vi "rainbow palette array.vi"() -> (0 "rainbow array":u32[](array[numeric]))   [LabVIEW 2009]
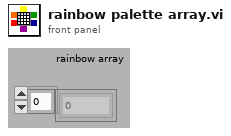
[diagram p1: front panel]
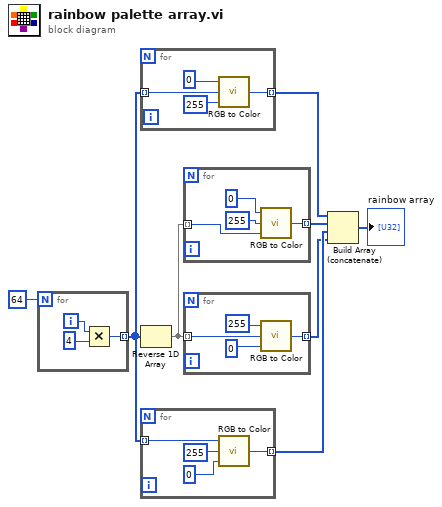
[diagram p0: block diagram]
diagram:
  n1 = for {
    N: 64 -> [_]
    tunnel: [w9] -> w7 mode=indexing
    i -> [w11]
    n2 = Multiply(x=w11, y=4) -> (x*y=w9:i32)
  }
  n3 = for {
    tunnel: w7 -> [w13] mode=indexing
    tunnel: [w12] -> w5 mode=indexing
    n4 = call <vilib>:"RGB to Color.vi"("B"=255, "G"=w13, "R"=0) -> ("Color"=w12:u32)
  }
  n5 = Reverse 1D Array(array=w7) -> (reversed array=w6:i32[])
  n6 = for {
    tunnel: [w19] -> w3 mode=indexing
    tunnel: w7 -> [w17] mode=indexing
    n7 = call <vilib>:"RGB to Color.vi"("B"=0, "G"=255, "R"=w17) -> ("Color"=w19:u32)
  }
  n8 = for {
    tunnel: [w22] -> w4 mode=indexing
    tunnel: w6 -> [w20] mode=indexing
    n9 = call <vilib>:"RGB to Color.vi"("B"=w20, "G"=255, "R"=0) -> ("Color"=w22:u32)
  }
  n10 = for {
    tunnel: [w27] -> w2 mode=indexing
    tunnel: w6 -> [w24] mode=indexing
    n11 = call <vilib>:"RGB to Color.vi"("B"=0, "G"=w24, "R"=255) -> ("Color"=w27:u32)
  }
  n12 = Build Array (concatenate)(w5, w4, w3, w2) -> (→"rainbow array":u32[])
